vi "Raw data Reader.vi"(5 "Num de tramas":u32, 6 "error in (no error)":errorcluster, 7 "Tamaño Script":i32, 8 "TRANSDUCTORES":u64, 9 "VISA Refnum in":refnum<visa-resource-name>) -> (0 "error out":errorcluster, 2 "Raw data":T1(array[cluster]), 3 "VISA reference":refnum<visa-resource-name>)   [LabVIEW 2014, in "CAP-USB.lvlib"]
uses:
  CAP-USB.lvlib
  1-Nivel/Enum S-M Reader.ctl
panel:
  out "read buffer":string
  out "Checksum OK?":bool
  in  "stop":bool
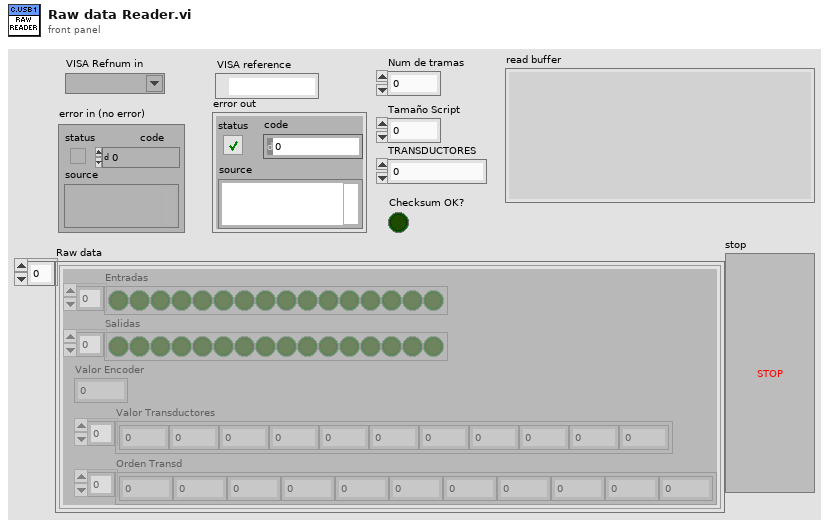
[diagram p1: front panel]
types:
  T1 = cluster{"Entradas":bool[], "Salidas":bool[], "Valor Encoder":u16, "Valor Transductores":u16[], "Orden Transd":u32[]}[]
  T2 = typedef "CAP-USB.lvlib/Enum S-M Reader.ctl" = enum16{"IDLE", "Detect 01"}
  T3 = cluster{"Entradas":bool[], "Salidas":bool[], "Valor Encoder":u16, "Valor Transductores":u16[], "Orden Transd":i32[]}
  T4 = cluster{"Entradas":bool[], "Salidas":bool[], "Valor Encoder":u16, "Valor Transductores":u16[], "Orden Transd":i32[]}[]
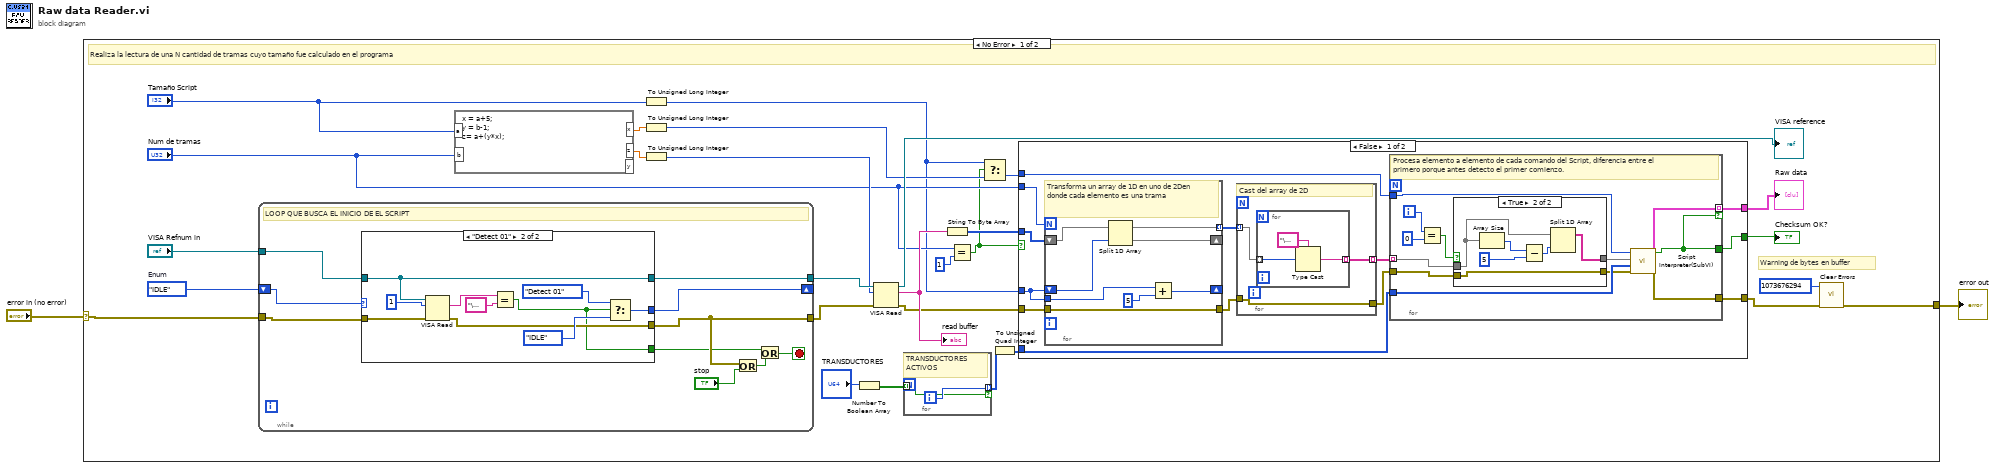
[diagram p0: block diagram]
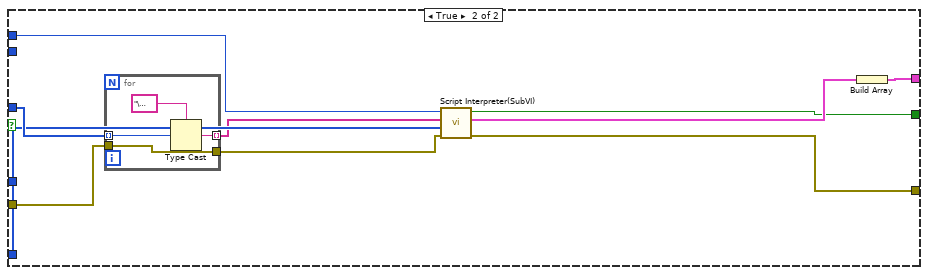
[diagram p3: hidden frame]
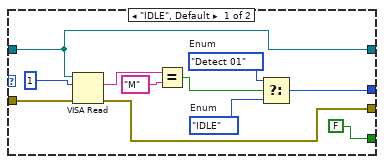
[diagram p4: hidden frame]
diagram:
  n1 = case shown="No Error" "error in (no error)" {
    selector: "error in (no error)" -> [w3 w125]
    tunnel: [w4 w125] -> w2
    frame No Error {
      w30 = Enum_S-M_Reader."IDLE"  # Enum
      # "Warning de bytes en buffer"
      # "Realiza la lectura de una N cantidad de tramas cuyo tamaño fue calculado en el programa"
      n2 = while {
        tunnel: "VISA Refnum in" -> [w103]
        tunnel: w3 -> [w102]
        shift-right: [w100] -> _
        shift-left: w30 -> [w101]
        tunnel: [w98] -> w28
        tunnel: [w97] -> w27
        stop <- w94 stop-if-true
        # "LOOP QUE BUSCA EL INICIO DE EL SCRIPT"
        n3 = case shown="\"Detect 01\"" w101 {
          tunnel: w103 -> [w105 w117]
          tunnel: w102 -> [w114 w118]
          tunnel: [w109 w120] -> w100
          tunnel: [FALSE w115] -> w95
          tunnel: [w105 w117] -> w98
          tunnel: [w104 w116] -> w97
          frame "IDLE", Default {
            w110 = Enum_S-M_Reader."IDLE"  # Enum
            w111 = Enum_S-M_Reader."Detect 01"  # Enum
            n4 = VISA Read(VISA resource name=w105, byte count=u32 1, error in (no error)=w114) -> (read buffer=w107:string, error out=w104:errorcluster)  [unwired: 2 out]
            n5 = Equal?(x=w107, y="M") -> (x = y?=w108:bool)
            n6 = Select(t=w111, s=w108, f=w110) -> (s? t:f=w109:T2)
          }
          frame "Detect 01" {
            n7 = VISA Read(VISA resource name=w117, byte count=u32 1, error in (no error)=w118) -> (read buffer=w119:string, error out=w116:errorcluster)  [unwired: 2 out]
            n8 = Equal?(x=w119, y="\u0001") -> (x = y?=w115:bool)
            n9 = Select(t=Enum_S-M_Reader."Detect 01" ("Enum"), s=w115, f=Enum_S-M_Reader."IDLE" ("Enum")) -> (s? t:f=w120:T2)
          }
        }
        n10 = Or(x=w97, y="stop") -> (x .or. y?=w96:bool)
        n11 = Or(x=w95, y=w96) -> (x .or. y?=w94:bool)
      }
      n12 = formula code="x = a+5;\ny = b-1;\nz= a+(y*x);"("a"="Tamaño Script", "b"="Num de tramas") -> ("x"=w15:dbl, "z"=w14:dbl)  [unwired: 1 out]
      n13 = To Unsigned Long Integer(number="Tamaño Script") -> (unsigned 32bit integer=w7:u32)
      n14 = To Unsigned Long Integer(number=w15) -> (unsigned 32bit integer=w10:u32)
      n15 = To Unsigned Long Integer(number=w14) -> (unsigned 32bit integer=w13:u32)
      n16 = Number To Boolean Array(number="TRANSDUCTORES") -> (Boolean array=w18:bool[])
      n17 = VISA Read(VISA resource name=w28, byte count=w13, error in (no error)=w27) -> (VISA resource name out=→"VISA reference":refnum<visa-resource-name>, read buffer=w24:string, error out=w23:errorcluster)  [unwired: 1 out]
      "read buffer" <- w24
      n18 = for {
        tunnel: w18 -> [w92] mode=indexing
        tunnel: [w93] -> w17 mode=indexing if=w92
        i -> [w93]
        # "TRANSDUCTORES\nACTIVOS"
      }
      n19 = String To Byte Array(string=w24) -> (unsigned byte array=w22:u8[])
      n20 = Equal?(x="Num de tramas", y=u32 1) -> (x = y?=w8:bool)
      n21 = Select(t=w7, s=w8, f=w10) -> (s? t:f=w9:u32)
      n22 = To Unsigned Quad Integer(1:w17) -> (0:w16:u64[])
      n23 = case shown="False" w8 {
        tunnel: [w43 w80] -> w25
        tunnel: [w42 w83] -> w5
        tunnel: w16 -> [w41 w86]
        tunnel: w7 -> [w39 _]
        tunnel: w23 -> [w38 w84]
        tunnel: w22 -> [w37 w87]
        tunnel: "Num de tramas" -> [w36 _]
        tunnel: [w32 w81] -> w21
        tunnel: w9 -> [w31 w79]
        frame False {
          n24 = for {
            N: w36 -> [_]
            shift-right: [w72] -> _
            shift-left: w37 -> [w74]
            shift-right: [w75] -> _
            shift-left: w39 -> [w73]
            tunnel: w39 -> [w77]
            tunnel: [w70] -> w40 mode=indexing
            tunnel: w38 -> [w71]
            tunnel: [w71] -> w34
            # "Transforma un array de 1D en uno de 2Den donde cada elemento es una trama"
            n25 = Split 1D Array(array=w74, index=w73) -> (first subarray=w70:u8[], second subarray=w72:u8[])
            n26 = Add(x=w77, y=u32 5) -> (x+y=w75:u32)
          }
          n27 = for {
            tunnel: w40 -> [w66] mode=indexing
            tunnel: [w65] -> w35 mode=indexing
            tunnel: w34 -> [w64]
            tunnel: [w64] -> w33
            # "Cast del array de 2D"
            n28 = for {
              tunnel: [w68] -> w65 mode=indexing
              tunnel: w66 -> [w67] mode=indexing
              n29 = Type Cast(type="\u0000", x=w67) -> (*(type *) &x=w68:string)
            }
          }
          n30 = for {
            tunnel: [w44] -> w43
            tunnel: [w55] -> w32 mode=indexing if=w44
            tunnel: [w54] -> w42
            tunnel: w41 -> [w53]
            tunnel: w31 -> [w52]
            tunnel: w35 -> [w48] mode=indexing
            tunnel: w33 -> [w47]
            i -> [w50]
            # "Procesa elemento a elemento de cada comando del Script, diferencia entre el primero porque antes detecto el primer comienzo."
            n31 = Equal?(x=w50, y=0) -> (x = y?=w51:bool)
            n32 = case shown="True" w51 {
              tunnel: w48 -> [w56 w58]
              tunnel: w47 -> [w57 w63]
              tunnel: [w57 w63] -> w46
              tunnel: [w56 w59] -> w45
              frame False {
              }
              frame True {
                n33 = Array Size(array=w58) -> (size(s)=w61:i32)
                n34 = Subtract(x=w61, y=5) -> (x-y=w62:i32)
                n35 = Split 1D Array(array=w58, index=w62) -> (first subarray=w59:string[])  [unwired: 1 out]
              }
            }
            n36 = call "Script Interpreter(SubVI).vi"("error in (no error)"=w46, "Transd IN"=w53, "Data IN"=w45, "Tamaño trama"=w52) -> ("error out"=w54:errorcluster, "Raw Data"=w55:T3, "Checksum"=w44:bool)  [unwired: 5 in]
          }
        }
        frame True {
          n37 = for {
            tunnel: [w90] -> w78 mode=indexing
            tunnel: w87 -> [w89] mode=indexing
            tunnel: [w88] -> w85
            tunnel: w84 -> [w88]
            n38 = Type Cast(type="\u0000", x=w89) -> (*(type *) &x=w90:string)
          }
          n39 = call "Script Interpreter(SubVI).vi"("error in (no error)"=w85, "Transd IN"=w86, "Data IN"=w78, "Tamaño trama"=w79) -> ("error out"=w83:errorcluster, "Raw Data"=w82:T3, "Checksum"=w80:bool)  [unwired: 5 in]
          n40 = Build Array(w82) -> (w81:T4)
        }
      }
      "Checksum OK?" <- w25
      "Raw data" <- w21
      n41 = call <vilib>:"Clear Errors.vi"("error in (no error)"=w5, "specific error code to clear (0: all)"=1073676294) -> ("error out"=w4:errorcluster)  [unwired: 4 in, 1 out]
    }
    frame Error {
    }
  }
  "error out" <- w2
